vi "Close.vi"(8 "error in (no error)":errorcluster, 11 "State in":T1={"State"=enum."Idle", "Start Time"=timestamp(0 s since 1904-01-01), "Configuration"={"Cycle Period"=0.0, "Manual Entry"=0.0, "Output Device"=enum."Ismatec ISM 831C", "Ismatech"={"VISA resource name"="", "Simulated?"=FALSE, "Pump Number"=1.0, "Reverse?"=FALSE}, "Ismatech 3 Channel Settings"={"VISA resource name"="", "Pump Number"=1, "Channel Number"=0, "Simulated?"=TRUE, "Reverse?"=FALSE}, "Masterflex"={"VISA resource name"="", "Simulated?"=FALSE, "Pump Number"=1.0, "Reverse?"=FALSE}, "VICI Settings"={"VISA resource name"="", "Pump ID"="", "Pump Head Vol"=0.0, "Reverse?"=FALSE, "Simulated?"=FALSE}, "Tacmina Settings"={"Analog DAQ Task"="", "Digital DAQ Task"=""}, "KNF SIMDOS Settings"={"VISA resource name"="", "Simulated?"=TRUE}, "ASIA Pump C"={"ASIA Pump #"=0, "channel"=0, "Simulated"=FALSE}, "FLOM Settings"={"VISA resource name"="", "Simulated?"=TRUE, "Pump Number"=0.0}, "SSI PR/LD Settings"={"VISA resource name"="", "Simulated?"=FALSE}, "SSI P40 Settings"={"VISA resource name"="", "Simulated?"=FALSE}, "Masterflex 75211 Settings"={"Analog DAQ Task"="", "Digital DAQ Task"=""}, "Pump Calibration File"=path "", "Calibration Slope"=0.0, "Calibration Y Intercept"=0.0, "Pump Cal Enum"=0, "Reset Totalizer"=FALSE}, "Current Time"=timestamp(0 s since 1904-01-01), "First Iteration"=FALSE, "Data"={"Pump Speed"=0.0, "Pump Pressure"=0.0, "Pump Flow"=0.0, "Totalized"=0.0}, "Process Name"="", "Pump On?"=enum."Off", "Output Error"=FALSE, "Log Started"=FALSE, "Overpressure Alarming"=FALSE} {"Configuration"."Ismatech 3 Channel Settings"."Channel Number" min=0 max=3; "Configuration"."Ismatech 3 Channel Settings"."Pump Number" min=1; "Configuration"."ASIA Pump C"."channel" min=0 max=1 step=1; "Configuration"."Masterflex"."Pump Number" min=1.0 max=20.0 step=1.0; "Configuration"."Ismatech"."Pump Number" min=1.0 max=20.0 step=1.0}) -> (0 "error out":errorcluster, 1 "Connection Error":bool, 3 "State out":T1={"State"=enum."Idle", "Start Time"=timestamp(0 s since 1904-01-01), "Configuration"={"Cycle Period"=0.0, "Manual Entry"=0.0, "Output Device"=enum."Ismatec ISM 831C", "Ismatech"={"VISA resource name"="", "Simulated?"=FALSE, "Pump Number"=1.0, "Reverse?"=FALSE}, "Ismatech 3 Channel Settings"={"VISA resource name"="", "Pump Number"=1, "Channel Number"=0, "Simulated?"=TRUE, "Reverse?"=FALSE}, "Masterflex"={"VISA resource name"="", "Simulated?"=FALSE, "Pump Number"=1.0, "Reverse?"=FALSE}, "VICI Settings"={"VISA resource name"="", "Pump ID"="", "Pump Head Vol"=0.0, "Reverse?"=FALSE, "Simulated?"=FALSE}, "Tacmina Settings"={"Analog DAQ Task"="", "Digital DAQ Task"=""}, "KNF SIMDOS Settings"={"VISA resource name"="", "Simulated?"=TRUE}, "ASIA Pump C"={"ASIA Pump #"=0, "channel"=0, "Simulated"=FALSE}, "FLOM Settings"={"VISA resource name"="", "Simulated?"=TRUE, "Pump Number"=0.0}, "SSI PR/LD Settings"={"VISA resource name"="", "Simulated?"=FALSE}, "SSI P40 Settings"={"VISA resource name"="", "Simulated?"=FALSE}, "Masterflex 75211 Settings"={"Analog DAQ Task"="", "Digital DAQ Task"=""}, "Pump Calibration File"=path "", "Calibration Slope"=0.0, "Calibration Y Intercept"=0.0, "Pump Cal Enum"=0, "Reset Totalizer"=FALSE}, "Current Time"=timestamp(0 s since 1904-01-01), "First Iteration"=FALSE, "Data"={"Pump Speed"=0.0, "Pump Pressure"=0.0, "Pump Flow"=0.0, "Totalized"=0.0}, "Process Name"="", "Pump On?"=enum."Off", "Output Error"=FALSE, "Log Started"=FALSE, "Overpressure Alarming"=FALSE} {"Configuration"."Ismatech 3 Channel Settings"."Channel Number" min=0 max=3; "Configuration"."Ismatech 3 Channel Settings"."Pump Number" min=1; "Configuration"."ASIA Pump C"."channel" min=0 max=1 step=1; "Configuration"."Masterflex"."Pump Number" min=1.0 max=20.0 step=1.0; "Configuration"."Ismatech"."Pump Number" min=1.0 max=20.0 step=1.0})   [LabVIEW 2018, in "Pump Module.lvlib" / "Pump Module Engine.lvlib"]
uses:
  Pump Module Engine.lvlib
  State Cluster.ctl
  State Enum.ctl
  Pump Module Settings Cluster.ctl
  Measure Instrument/PID 2 Output Enum.ctl
  Ismatec ISM 831C/Controls/Ismatech ISM831C Settings Cluster.ctl
  Ismatec 78001/Ismatec 4083.ctl
  Masterflex 7550-30/Controls/Settings Cluster.ctl
  VICI M50 Party Mode/Settings Cluster.ctl
  Tacmina QI/Tacmina QI DAQ Setting.ctl
  KNF Pump/Settings Cluster plus SIMDOS.ctl
  ASIA Pump/Pump Settings.ctl
  FLOM Pump/Settings Cluster.ctl
  SSI PR Class/SSI PR or LD Settings Cluster.ctl
  Masterflex 75211/Masterflex 75211 DAQ Setting.ctl
  Tag VIs/Tag FGV Operation Enum.ctl
  Masterflex 7550-30/Masterflex 7550-30.lvlib
  Ismatec ISM 831C/Ismatec ISM 831C.lvlib
  Tacmina QI/Tacmina QI.lvlib
  VICI M50 Party Mode/VICI M6 M50 Party Mode.lvlib
  ASIA Pump.lvlib
  KNF Pump/KNF SIMDOS.lvlib
  FLOM Pump/FLOM Pump.lvlib
  SSI PR Class/SSI PR or LD Pump.lvlib
  Shared Variables/Dynamic Shared Variables.lvlib
  Masterflex 75211/Masterflex 75211.lvlib
  SSI PR Class/SSI P40 Pump.lvlib
  Ismatec 78001/Ismatec 4308.lvlib
  Pump Module.lvlib
panel:
  # "Output Instruments"
  # "Output Instruments"
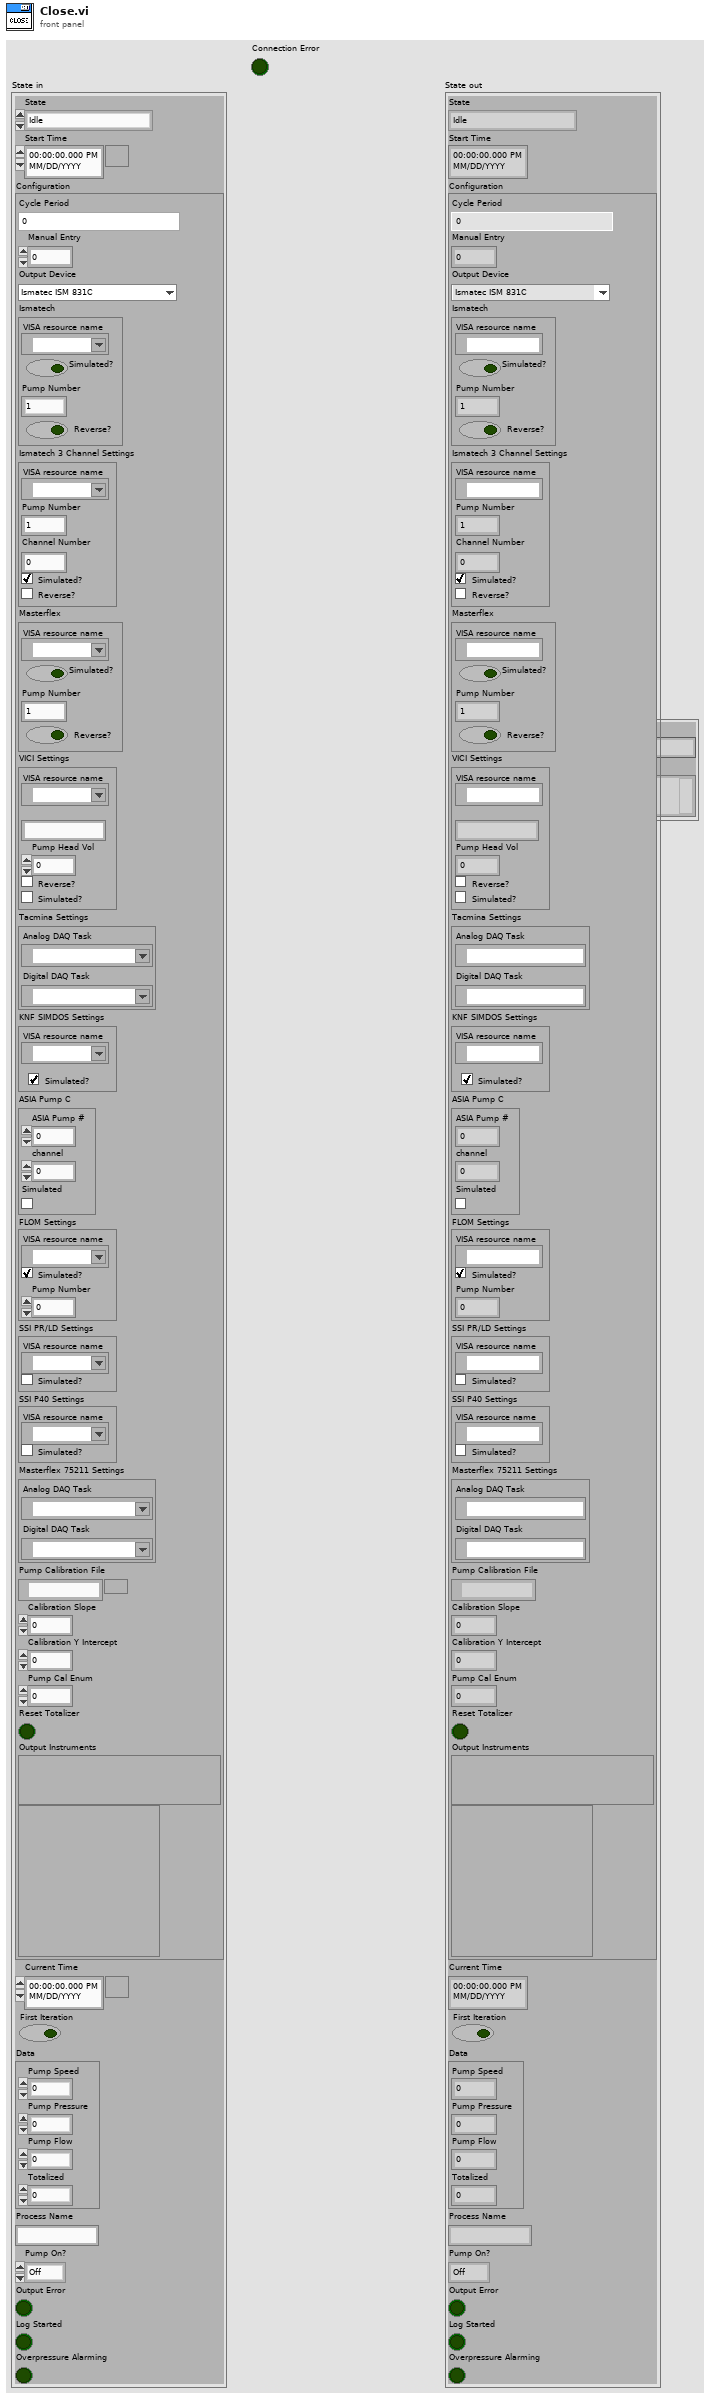
[diagram p1: front panel]
types:
  T1 = typedef "Pump Module.lvlib/Pump Module Engine.lvlib/State Cluster.ctl" = cluster{"State":T2, "Start Time":timestamp, "Configuration":T3, "Current Time":timestamp, "First Iteration":bool, "Data":cluster{"Pump Speed":dbl, "Pump Pressure":dbl, "Pump Flow":dbl, "Totalized":dbl}, "Process Name":string, "Pump On?":enum16{"Off", "On", "Not Initialized"}, "Output Error":bool, "Log Started":bool, "Overpressure Alarming":bool}
  T2 = typedef "Pump Module.lvlib/Pump Module Engine.lvlib/State Enum.ctl" = enum16{"Measuring", "Idle", "Paused"}
  T3 = typedef "Pump Module.lvlib/Pump Module Settings Cluster.ctl" = cluster{"Cycle Period":dbl, "Manual Entry":dbl, "Output Device":T4, "Ismatech":T5, "Ismatech 3 Channel Settings":T6, "Masterflex":T7, "VICI Settings":T8, "Tacmina Settings":T9, "KNF SIMDOS Settings":T10, "ASIA Pump C":T11, "FLOM Settings":T12, "SSI PR/LD Settings":T13, "SSI P40 Settings":T13, "Masterflex 75211 Settings":T14, "Pump Calibration File":path, "Calibration Slope":dbl, "Calibration Y Intercept":dbl, "Pump Cal Enum":u16, "Reset Totalizer":bool}
  T4 = typedef "PID 2 Output Enum.ctl" = enum16{"Default", "Ismatec ISM 4308", "Ismatec ISM 831C", "Masterflex 7550-30", "VICI M6", "VICI M50", "Tacmina QI", "KNF SIMDOS", "ASIA Type C", "FLOM UI-22-11", "SSI PR/LD", "SSI P40", "Masterflex 75211-70"}
  T5 = typedef "Ismatec ISM 831C.lvlib/Ismatech ISM831C Settings Cluster.ctl" = cluster{"VISA resource name":refnum<visa-resource-name>, "Simulated?":bool, "Pump Number":dbl, "Reverse?":bool}
  T6 = typedef "Ismatec 4308.lvlib/Ismatec 4083.ctl" = cluster{"VISA resource name":refnum<visa-resource-name>, "Pump Number":i16, "Channel Number":i16, "Simulated?":bool, "Reverse?":bool}
  T7 = typedef "Masterflex 7550-30.lvlib/Settings Cluster.ctl" = cluster{"VISA resource name":refnum<visa-resource-name>, "Simulated?":bool, "Pump Number":dbl, "Reverse?":bool}
  T8 = typedef "VICI M6 M50 Party Mode.lvlib/Settings Cluster.ctl" = cluster{"VISA resource name":refnum<visa-resource-name>, "Pump ID":string, "Pump Head Vol":dbl, "Reverse?":bool, "Simulated?":bool}
  T9 = typedef "Tacmina QI.lvlib/Tacmina QI DAQ Setting.ctl" = cluster{"Analog DAQ Task":refnum<k21>, "Digital DAQ Task":refnum<k21>}
  T10 = typedef "KNF SIMDOS.lvlib/Settings Cluster plus SIMDOS.ctl" = cluster{"VISA resource name":refnum<visa-resource-name>, "Simulated?":bool}
  T11 = typedef "ASIA Pump.lvlib/Pump Settings.ctl" = cluster{"ASIA Pump #":i32, "channel":i32, "Simulated":bool}
  T12 = typedef "FLOM Pump.lvlib/Settings Cluster.ctl" = cluster{"VISA resource name":refnum<visa-resource-name>, "Simulated?":bool, "Pump Number":dbl}
  T13 = typedef "SSI PR or LD Pump.lvlib/SSI PR or LD Settings Cluster.ctl" = cluster{"VISA resource name":refnum<visa-resource-name>, "Simulated?":bool}
  T14 = typedef "Masterflex 75211.lvlib/Masterflex 75211 DAQ Setting.ctl" = cluster{"Analog DAQ Task":refnum<k21>, "Digital DAQ Task":refnum<k21>}
  T15 = typedef "Pump Module.lvlib/Pump Module Tag Names Cluster.ctl" = cluster{"Pump Speed":string, "Totalized g Tag":string, "Pump Flow":string, "Pump Pressure":string, "Output Device Tag":string, "Overpressure Tag":string, "Identifier Tag":string}
  T16 = typedef "SSI P40 Pump.lvlib/SSI P40 Settings Cluster.ctl" = cluster{"VISA resource name":refnum<visa-resource-name>, "Simulated?":bool}
  T17 = typedef "Tag FGV Operation Enum.ctl" = enum16{"Init", "Set Notification Queue", "Create Tag", "Commit", "Write Tag (Numeric)", "Write Tag (Boolean)", "Read All Tags", "Read One Tag", "Delete Tag Category", "Set Alarm Parameters (Numeric)", "Set Alarm Parameters (Boolean)", "Enable All Alarms", "Disable All Alarms", "Delete All Tags", "Read Alarms", "Ack Alarm", "Read Alarm Parameters (Numeric)", "Read Alarm Parameters (Boolean)"}
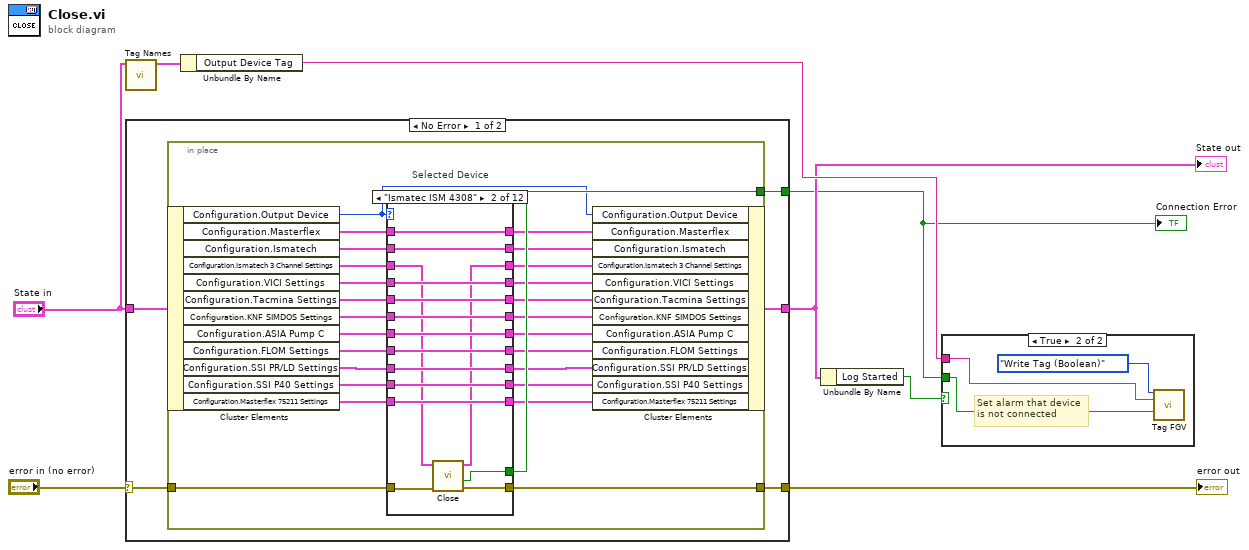
[diagram p0: block diagram]
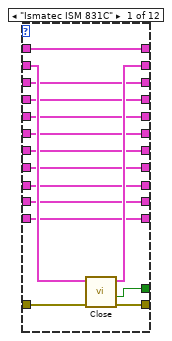
[diagram p3: hidden frame]
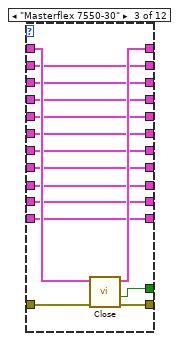
[diagram p4: hidden frame]
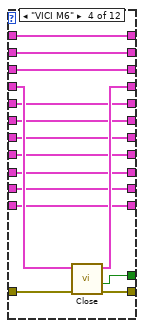
[diagram p5: hidden frame]
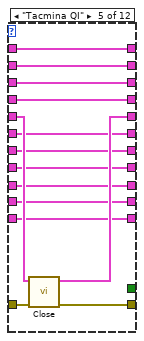
[diagram p6: hidden frame]
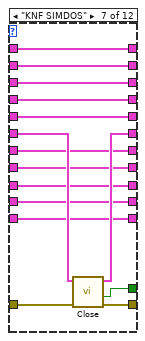
[diagram p8: hidden frame]
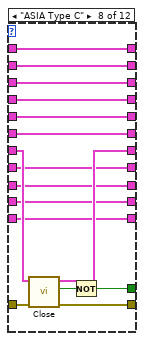
[diagram p9: hidden frame]
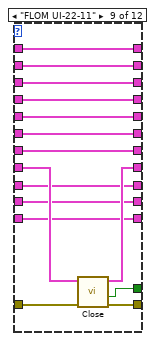
[diagram p10: hidden frame]
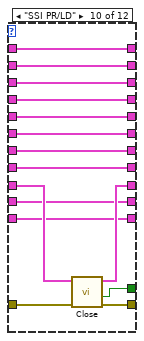
[diagram p11: hidden frame]
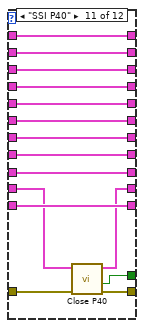
[diagram p12: hidden frame]
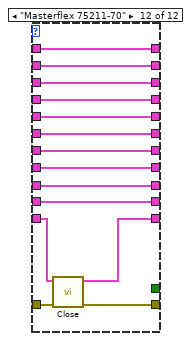
[diagram p13: hidden frame]
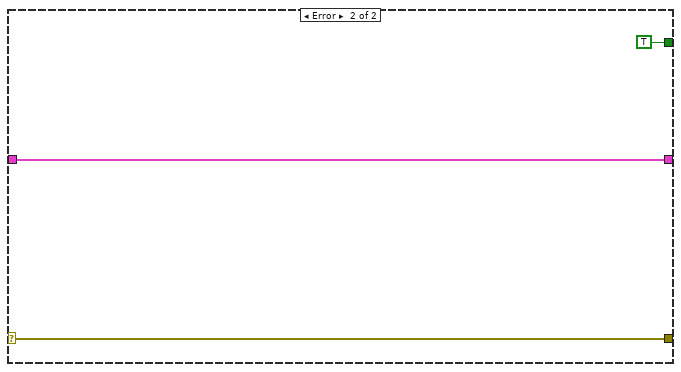
[diagram p14: hidden frame]
diagram:
  n1 = call "Tag Names.vi"("State In"="State in") -> ("Pump Module Tag Names"=w5:T15)  [unwired: 8 in, 2 out]
  n2 = case shown="No Error" "error in (no error)" {
    selector: "error in (no error)" -> [w12 w218]
    tunnel: [w13 w218] -> w7
    tunnel: "State in" -> [w10 w217]
    tunnel: [w9 w217] -> w3
    tunnel: [w11 TRUE ("Connection Error")] -> w1
    frame No Error {
      n3 = in-place {
        in-place-border: [w39] -> w13
        in-place-border: w12 -> [w38]
        in-place-border: [w37] -> w11
        n4 = in-place-cluster #1(w10) -> ("Configuration.Output Device"=w19:T4, "Configuration.Masterflex"=w36:T7, "Configuration.Ismatech"=w35:T5, "Configuration.Ismatech 3 Channel Settings"=w14:T6, "Configuration.VICI Settings"=w34:T8, "Configuration.Tacmina Settings"=w33:T9, "Configuration.KNF SIMDOS Settings"=w32:T10, "Configuration.ASIA Pump C"=w31:T11, "Configuration.FLOM Settings"=w30:T12, "Configuration.SSI PR/LD Settings"=w29:T13, "Configuration.SSI P40 Settings"=w17:T13, "Configuration.Masterflex 75211 Settings"=w20:T14)
        n5 = case "Selected Device" shown="\"Ismatec ISM 4308\"" w19 {
          tunnel: w36 -> [w50 w69 w84 w94 w110 w125 w136 w154 w171 w186 w201 w215]
          tunnel: [w50 w69 w83 w94 w110 w125 w136 w154 w171 w186 w201 w215] -> w28
          tunnel: w35 -> [w52 w60 w81 w95 w111 w121 w135 w153 w170 w185 w200 w214]
          tunnel: [w54 w56 w82 w97 w112 w124 w139 w155 w164 w178 w191 w206] -> w39
          tunnel: w38 -> [w53 w55 w80 w98 w113 w124 w140 w156 w165 w179 w192 w207]
          tunnel: [w51 w60 w81 w95 w111 w121 w135 w153 w170 w185 w200 w214] -> w27
          tunnel: w34 -> [w49 w68 w79 w99 w108 w123 w134 w152 w169 w184 w199 w213]
          tunnel: [w49 w68 w79 w96 w108 w123 w134 w152 w169 w184 w199 w213] -> w26
          tunnel: w33 -> [w48 w67 w78 w93 w107 w122 w133 w151 w168 w183 w198 w212]
          tunnel: [w48 w67 w78 w93 w109 w122 w133 w151 w168 w183 w198 w212] -> w25
          tunnel: w32 -> [w47 w66 w77 w91 w106 w119 w138 w150 w167 w182 w197 w211]
          tunnel: [w47 w66 w77 w91 w106 w119 w137 w150 w167 w182 w197 w211] -> w24
          tunnel: [w46 w65 w76 w92 w105 w120 w132 w148 w166 w181 w196 w210] -> w23
          tunnel: w31 -> [w46 w65 w76 w92 w105 w120 w132 w149 w166 w181 w196 w210]
          tunnel: w30 -> [w45 w64 w75 w90 w104 w118 w131 w147 w163 w180 w195 w209]
          tunnel: [w45 w64 w75 w90 w104 w118 w131 w147 w162 w180 w195 w209] -> w22
          tunnel: w29 -> [w44 w63 w74 w89 w103 w117 w130 w146 w161 w177 w194 w208]
          tunnel: [w44 w63 w74 w89 w103 w117 w130 w146 w161 w176 w194 w208] -> w21
          tunnel: [w43 w57 w73 w88 _ _ w129 w144 w160 w175 w190 _] -> w37
          tunnel: w20 -> [w42 w62 w72 w87 w102 w116 w128 w143 w159 w174 w193 w205]
          tunnel: [w42 w62 w72 w87 w102 w116 w128 w143 w159 w174 w193 w204] -> w18
          tunnel: w17 -> [w41 w61 w71 w86 w101 w115 w127 w142 w158 w173 w188 w203]
          tunnel: [w41 w61 w71 w86 w101 w115 w127 w142 w158 w173 w189 w203] -> w16
          tunnel: [w40 w58 w70 w85 w100 w114 w126 w141 w157 w172 w187 w202] -> w15
          tunnel: w14 -> [w40 w59 w70 w85 w100 w114 w126 w141 w157 w172 w187 w202]
          frame "Ismatec ISM 831C" {
            n6 = call "Close.vi"("error in (no error)"=w53, "Ismatech Settings"=w52) -> ("error out"=w54:errorcluster, "Connection Error"=w43:bool, "Ismatech Settings"=w51:T5)  [unwired: 7 in]
          }
          frame "Ismatec ISM 4308" {
            n7 = call "Close.vi"("error in (no error)"=w55, "Ismatech 3 Channel Settings In"=w59) -> ("error out"=w56:errorcluster, "Connection Error"=w57:bool, "Ismatech 3 Channel Settings Out"=w58:T6)  [unwired: 7 in]
          }
          frame "Masterflex 7550-30" {
            n8 = call "Close.vi"("error in (no error)"=w80, "Masterflex Settings in"=w84) -> ("error out"=w82:errorcluster, "Connection Error"=w73:bool, "Masterflex Settings out"=w83:T7)  [unwired: 7 in]
          }
          frame "VICI M6" {
            n9 = call "Close.vi"("error in (no error)"=w98, "VICI Settings"=w99) -> ("error out"=w97:errorcluster, "Connection Error"=w88:bool, "VICI Settings"=w96:T8)  [unwired: 7 in]
          }
          frame "Tacmina QI" {
            n10 = call "Close.vi"("error in"=w113, "Tacmina Settings in"=w107) -> ("error out"=w112:errorcluster, "Tacmina Settings out"=w109:T9)  [unwired: 8 in]
          }
          frame "Default", Default {
          }
          frame "KNF SIMDOS" {
            n11 = call "Close.vi"("error in (no error)"=w140, "KNF Settings"=w138) -> ("error out"=w139:errorcluster, "Connection Error"=w129:bool, "KNF Settings"=w137:T10)  [unwired: 7 in]
          }
          frame "ASIA Type C" {
            n12 = call "Close.vi"("error in (no error)"=w156, "ASIA Pump C"=w149) -> ("error out"=w155:errorcluster, "Task Completed"=w145:bool, "ASIA Pump C"=w148:T11)  [unwired: 7 in]
            n13 = Not(x=w145) -> (.not. x?=w144:bool)
          }
          frame "FLOM UI-22-11" {
            n14 = call "Close.vi"("error in (no error)"=w165, "FLOM Settings in"=w163) -> ("error out"=w164:errorcluster, "Connection Error"=w160:bool, "FLOM Settings out"=w162:T12)  [unwired: 7 in]
          }
          frame "SSI PR/LD" {
            n15 = call "Close.vi"("error in (no error)"=w179, "SSI PR Settings In"=w177) -> ("error out"=w178:errorcluster, "Connection Error"=w175:bool, "SSI PR Settings Out"=w176:T13)  [unwired: 7 in]
          }
          frame "SSI P40" {
            n16 = call "Close P40.vi"("error in (no error)"=w192, "SSI P40 Settings In"=w188) -> ("error out"=w191:errorcluster, "Connection Error"=w190:bool, "SSI P40 Settings Out"=w189:T16)  [unwired: 7 in]
          }
          frame "Masterflex 75211-70" {
            n17 = call "Close.vi"("error in"=w207, "Masterflex 75211 Settings"=w205) -> ("error out"=w206:errorcluster, "Masterflex 75211 Settings"=w204:T14)  [unwired: 8 in]
          }
        }
        n18 = in-place-cluster #1("Configuration.Output Device"=w19, "Configuration.Masterflex"=w28, "Configuration.Ismatech"=w27, "Configuration.Ismatech 3 Channel Settings"=w15, "Configuration.VICI Settings"=w26, "Configuration.Tacmina Settings"=w25, "Configuration.KNF SIMDOS Settings"=w24, "Configuration.ASIA Pump C"=w23, "Configuration.FLOM Settings"=w22, "Configuration.SSI PR/LD Settings"=w21, "Configuration.SSI P40 Settings"=w16, "Configuration.Masterflex 75211 Settings"=w18) -> (w9:T1)
      }
    }
    frame Error {
    }
  }
  "error out" <- w7
  "State out" <- w3
  "Connection Error" <- w1
  n19 = Unbundle By Name(w5) -> ("Output Device Tag"=w6:string)
  n20 = Unbundle By Name(w3) -> ("Log Started"=w2:bool)
  n21 = case shown="True" w2 {
    tunnel: w6 -> [_ w221]
    tunnel: w1 -> [_ w219]
    frame False {
    }
    frame True {
      # "Set alarm that device\nis not connected"
      n22 = call "Tag FGV.vi"("Operation"=Tag_FGV_Operation_Enum."Write Tag (Boolean)", "Tag Name"=w221, "Data"=w219) -> ()  [unwired: 5 in, 8 out]
    }
  }
